vi "Eject USB drives (SubVI).vi"(8 "error in (no error)":errorcluster, 11 "USB drive's list":path[](array[path])) -> (0 "error out":errorcluster)   [LabVIEW 2018]
uses:
  System.Management.Automation
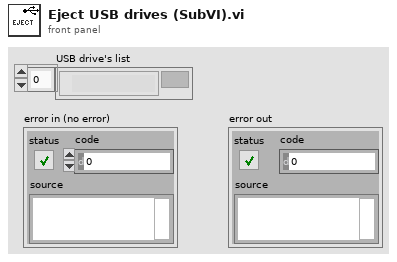
[diagram p1: front panel]
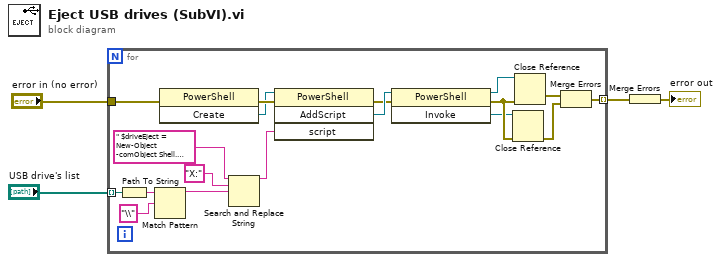
[diagram p0: block diagram]
diagram:
  n1 = for {
    tunnel: "USB drive's list" -> [w22] mode=indexing
    tunnel: [w6] -> w4 mode=indexing
    tunnel: "error in (no error)" -> [w5]
    n2 = Path To String(path=w22) -> (string=w20:string)
    n3 = Match Pattern(string=w20, regular expression="\\") -> (before substring=w17:string)  [unwired: 1 in, 3 out]
    n4 = invoke class="PowerShell" method="Create"(error in=w5) -> (error out=w13:errorcluster, "Create"=w10:refnum<k24>)  [unwired: 2 in, 1 out]
    n5 = Search and Replace String(input string=" $driveEject = New-Object -comObject Shell.Application\n$driveEject.Namespace(17).ParseName(\"X:\").InvokeVerb(\"Eject\")", search string="X:", replace string=w17) -> (result string=w9:string)  [unwired: 5 in, 3 out]
    n6 = invoke class="PowerShell" method="AddScript"(reference=w10, error in=w13, "script"=w9) -> (error out=w14:errorcluster, "AddScript"=w15:refnum<k24>)  [unwired: 1 in, 2 out]
    n7 = invoke class="PowerShell" method="Invoke"(reference=w15, error in=w14) -> (reference out=w12:refnum<k24>, error out=w16:errorcluster, "Invoke"=w11:refnum<k24>)  [unwired: 1 in]
    n8 = Close Reference(reference=w11, error in (no error)=w16) -> (error out=w8:errorcluster)
    n9 = Close Reference(reference=w12, error in (no error)=w16) -> (error out=w7:errorcluster)
    n10 = Merge Errors(w7, w8) -> (w6:errorcluster)
  }
  n11 = Merge Errors(w4) -> (→"error out":errorcluster)
